vi "move rotate speed.vi"(0 "rotate degree":dbl, 5 "now degree 2":dbl, 7 "i":i32, 9 "speed":dbl, 11 "dt(s)":dbl, 12 "t3 in":dbl) -> (3 "speed":dbl, 4 "speed out":dbl[](array[numeric]), 6 "deg(defference)":dbl, 8 "t2":dbl, 10 "t2?":bool, 14 "t3":dbl, 15 "complet?":bool)   [LabVIEW 2019]
panel:
  out "Numeric 2":dbl
  in  "Numeric":dbl
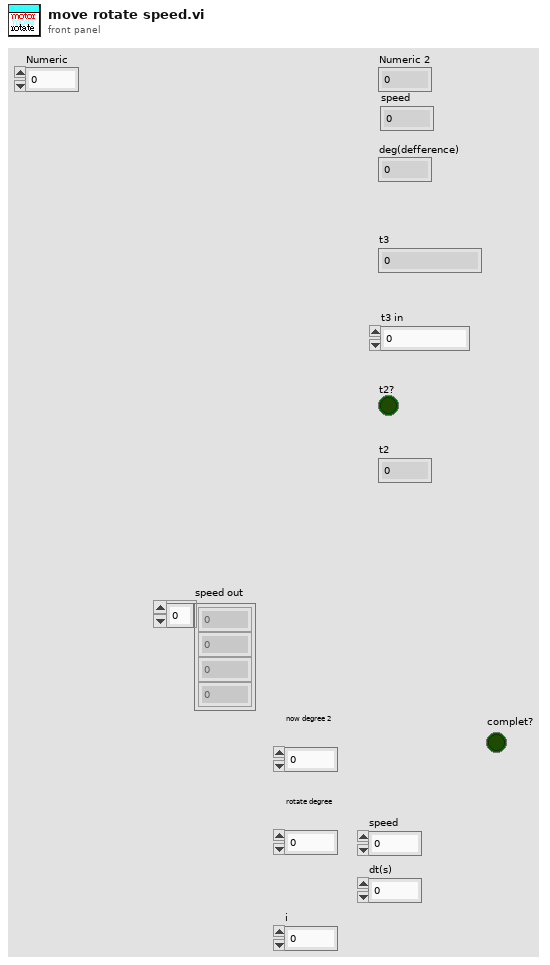
[diagram p1: front panel]
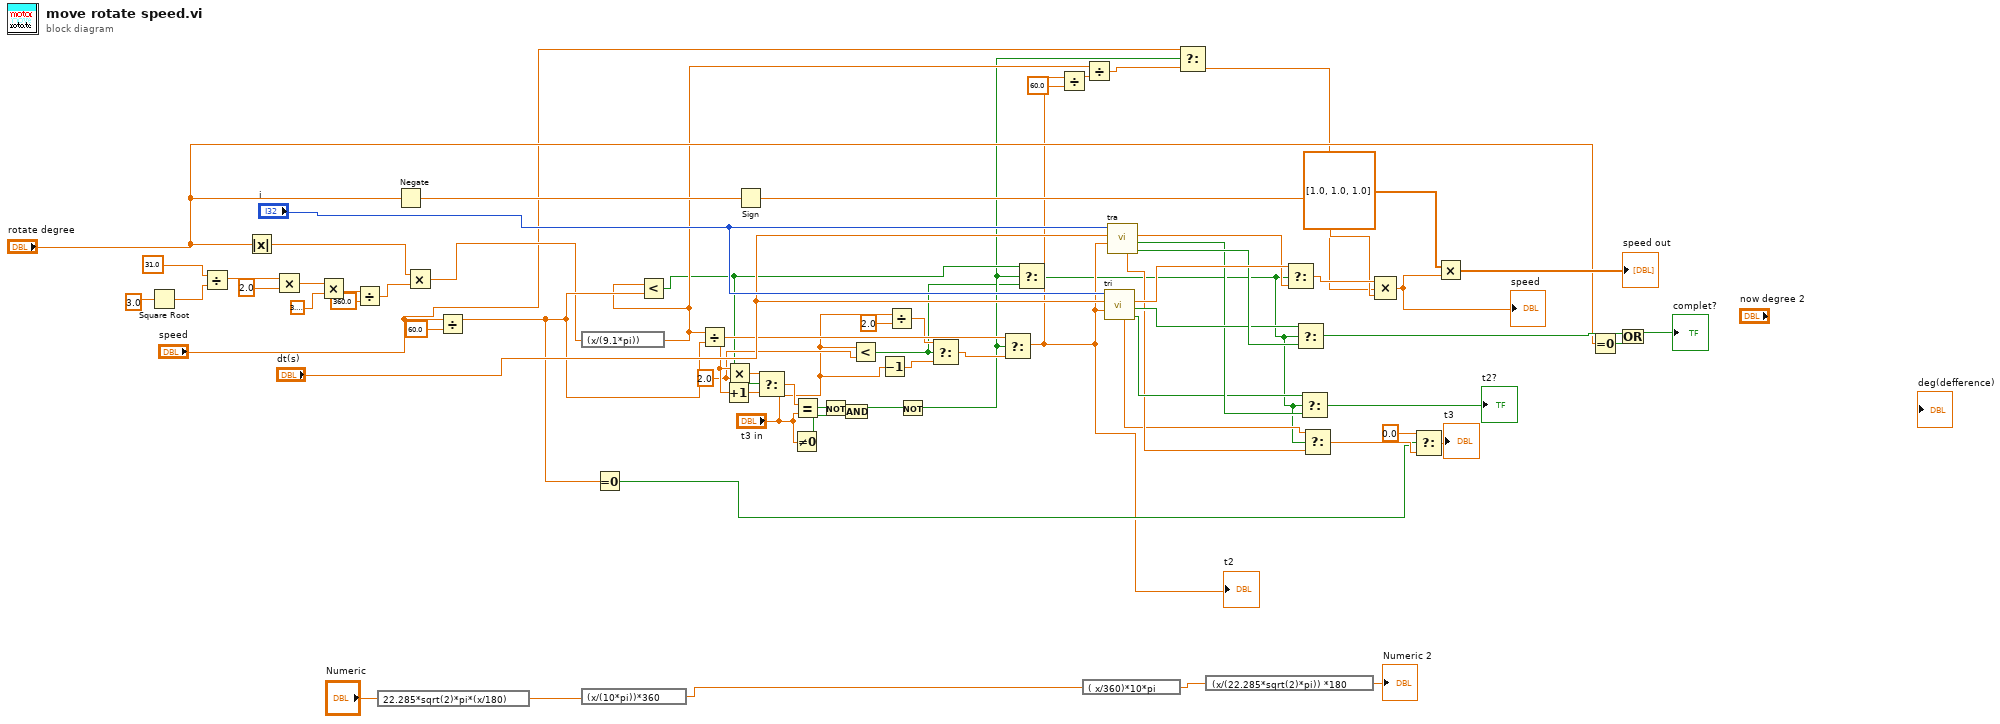
[diagram p0: block diagram]
diagram:
  w15 = 2.0 ("y")
  n1 = Square Root(x=3.0) -> (sqrt(x)=w38:dbl)
  n2 = Divide(x=31.0, y=w38) -> (x/y=w36:dbl)
  n3 = Absolute Value(x="rotate degree") -> (abs(x)=w30:dbl)
  n4 = Multiply(x=w36, y=2.0) -> (x*y=w33:dbl)
  n5 = Multiply(x=w33, y=3.141592653589793) -> (x*y=w32:dbl)
  n6 = Divide(x=w32, y=360.0) -> (x/y=w29:dbl)
  n7 = expression code="22.285*sqrt(2)*pi*(x/180)"("Numeric") -> (w51:dbl)
  n8 = Negate(x="rotate degree") -> (-x=w43:dbl)
  n9 = Multiply(x=w30, y=w29) -> (x*y=w28:dbl)
  n10 = Divide(x="speed", y=60.0) -> (x/y=w44:dbl)
  n11 = expression code="(x/(9.1*pi))"(w28) -> (w10:dbl)
  n12 = expression code="(x/(10*pi))*360"(w51) -> (w50:dbl)
  n13 = Equal To 0?(x=w44) -> (x = 0?=w59:bool)
  n14 = Less?(x=w10, y=w44) -> (x < y?=w3:bool)
  n15 = Divide(x=w10, y=w44) -> (x/y=w23:dbl)
  n16 = Increment(x=w23) -> (x+1=w24:dbl)
  n17 = Multiply(x=w23, y=w15) -> (x*y=w25:dbl)
  n18 = Sign(1:w43) -> (0:w47:dbl)
  n19 = Select(t=w25, s=w3, f=w24) -> (s? t:f=w22:dbl)
  n20 = Not Equal To 0?(x="t3 in") -> (x != 0?=w17:bool)
  n21 = Equal?(x=w22, y="t3 in") -> (x = y?=w19:bool)
  n22 = Not(x=w19) -> (.not. x?=w8:bool)
  n23 = And(x=w8, y=w17) -> (x .and. y?=w18:bool)
  n24 = Less?(x="t3 in", y=w15) -> (x < y?=w1:bool)
  n25 = Decrement(x="t3 in") -> (x-1=w13:dbl)
  n26 = Divide(x="t3 in", y=2.0) -> (x/y=w16:dbl)
  n27 = Not(x=w18) -> (.not. x?=w2:bool)
  n28 = Select(t=w16, s=w1, f=w13) -> (s? t:f=w11:dbl)
  n29 = Select(t=w23, s=w2, f=w11) -> (s? t:f=w9:dbl)
  "t2" <- w9
  n30 = Select(t=w3, s=w2, f=w1) -> (s? t:f=w4:bool)
  n31 = Divide(x=w9, y=60.0) -> (x/y=w6:dbl)
  n32 = expression code="( x/360)*10*pi"(w50) -> (w52:dbl)
  n33 = Divide(x=w10, y=w6) -> (x/y=w7:dbl)
  n34 = call "tri.vi"("t2"=w9, "dt(s)"="dt(s)", "i"="i") -> ("t2?"=w63:bool, "complet?"=w66:bool, "Waveform Chart"=w69:dbl, "t3"=w27:dbl)  [unwired: 5 in]
  n35 = call "tra.vi"("t2"=w9, "dt(s)"="dt(s)", "i"="i") -> ("complet?"=w67:bool, "t2?"=w64:bool, "Waveform Chart"=w68:dbl, "t3"=w62:dbl)  [unwired: 4 in, 1 out]
  n36 = Select(t="speed", s=w2, f=w7) -> (s? t:f=w21:dbl)
  n37 = expression code="(x/(22.285*sqrt(2)*pi)) *180"(w52) -> (→"Numeric 2":dbl)
  n38 = Select(t=w69, s=w4, f=w68) -> (s? t:f=w65:dbl)
  n39 = Select(t=w66, s=w4, f=w67) -> (s? t:f=w46:bool)
  n40 = Select(t=w63, s=w4, f=w64) -> (s? t:f=→"t2?":bool)
  n41 = Select(t=w27, s=w4, f=w62) -> (s? t:f=w61:dbl)
  n42 = Compound Arithmetic op=MULTIPLY(w65, w21, w47) -> (w54:dbl)
  "speed" <- w54
  n43 = Select(t=0.0, s=w59, f=w61) -> (s? t:f=→"t3":dbl)
  n44 = Multiply(x=dbl[] [1.0, 1.0, 1.0], y=w54) -> (x*y=→"speed out":dbl[])
  n45 = Equal To 0?(x="rotate degree") -> (x = 0?=w41:bool)
  n46 = Or(x=w46, y=w41) -> (x .or. y?=→"complet?":bool)
